vi "get_component_specification.vi"(8 "error in (no error)":errorcluster, 11 "StreamingBase in":refnum<class "StreamingBase.lvclass">) -> (0 "error out":errorcluster, 2 "component specification":T1, 3 "StreamingBase out":refnum<class "StreamingBase.lvclass">)   [LabVIEW 2011, in "StreamingBase.lvclass"]
uses:
  StreamingBase.lvclass
  component_specification_cluster.ctl
  StreamingBase.lvclass/StreamingBase.ctl
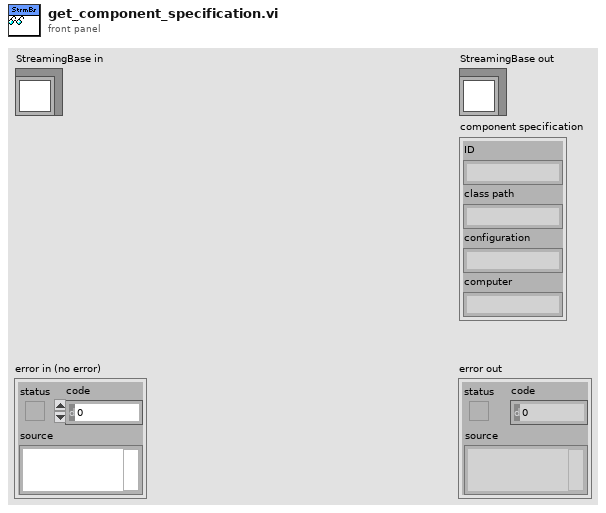
[diagram p1: front panel]
types:
  T1 = typedef "StreamingBase.lvclass/component_specification_cluster.ctl" = cluster{"ID":string, "class path":string, "configuration":string, "computer":string}
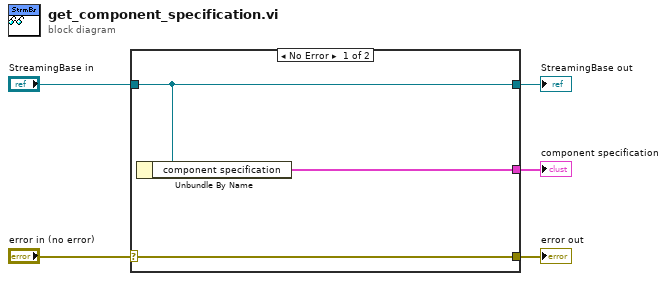
[diagram p0: block diagram]
diagram:
  n1 = case shown="No Error" "error in (no error)" {
    selector: "error in (no error)" -> [w8 w9]
    tunnel: [w8 w9] -> w4
    tunnel: [w7 w10] -> w2
    tunnel: "StreamingBase in" -> [w7 w10]
    tunnel: [w6 _] -> w1
    frame No Error {
      n2 = Unbundle By Name(w7) -> ("component specification"=w6:T1)
    }
    frame Error {
    }
  }
  "error out" <- w4
  "StreamingBase out" <- w2
  "component specification" <- w1
